vi "Reset Composite Limit Test.vi"(8 "error in (no error)":errorcluster, 10 "Channel (0: Channel 1)":i32(ring) items=["Channel 1", "Channel 2"], 11 "VISA resource name":refnum<visa-resource-name>) -> (0 "error out":errorcluster, 3 "VISA resource name out":refnum<visa-resource-name>)   [LabVIEW 2020, in "Agilent B2900 Series.lvlib"]
doc: "Clears the composite limit test results and the GPIO lines immediately.\n\n<B>Note:</B>\n(1) Use this VI only with other low-level VIs. The high-level VIs automatically incorporate this functionality. This VI does not check the instrument status. \n(2) This VI is not applicable for Agilent models B2961A, B2962A, B2961B, B2962B, B2961C and B2962C."
uses:
  Agilent B2900 Series.lvlib
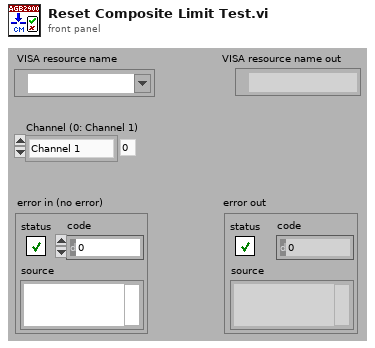
[diagram p1: front panel]
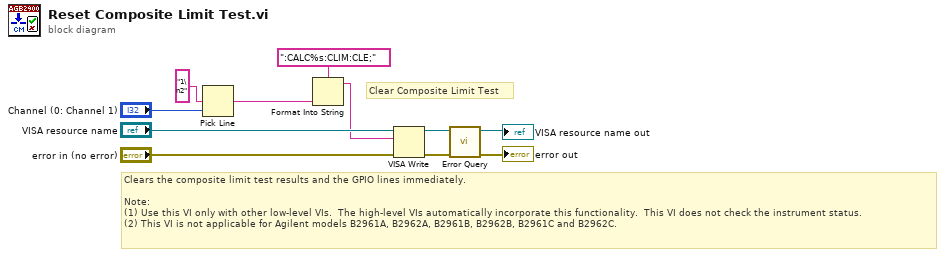
[diagram p0: block diagram]
diagram:
  # "Clears the composite limit test results and the GPIO lines immediately.\n\nNote:\n(1) Use this VI only with other low-level VIs.  The high-level VIs automatically incorporate this functionality.  This VI does not check the instrument status.   \n(2) This VI is not applicable for Agilent models B2961A, B2962A, B2961B, B2962B, B2961C and B2962C."
  # "Clear Composite Limit Test"
  n1 = Pick Line(multi-line string="1\n2" ("string (\"\")"), line index="Channel (0: Channel 1)") -> (output string=w6:string)  [unwired: 1 in]
  n2 = Format Into String(format string=":CALC%s:CLIM:CLE;", w6) -> (resulting string=w5:string)  [unwired: 2 in, 1 out]
  n3 = VISA Write(VISA resource name="VISA resource name", write buffer=w5, error in (no error)="error in (no error)") -> (VISA resource name out=w2:refnum<visa-resource-name>, error out=w1:errorcluster)  [unwired: 1 out]
  n4 = call "Error Query.vi"("error in (no error)"=w1, "VISA resource name"=w2) -> ("error out"=→"error out":errorcluster, "VISA resource name out"=→"VISA resource name out":refnum<visa-resource-name>)  [unwired: 6 in, 2 out]
